vi "Execution Settings.vi"(8 "error in (no error)":errorcluster, 11 "Configuration in":refnum<class "Configuration.lvclass">) -> (0 "error out":errorcluster, 3 "Configuration out":refnum<class "Configuration.lvclass">)   [LabVIEW 2026, in "Measurement Actor.lvlib" / "Step Configuration.lvclass"]
uses:
  Step Configuration.lvclass
  Extensible-Config-Dialog/Configuration.lvclass
  C:/Users/E2013170/Documents/GitHub/Measurement-Utility-Reference/components/Extensible-Config-Dialog/Configuration.lvclass
  Step Configuration.lvclass/Step Configuration.ctl
panel:
  in  "Execution Settings":T1
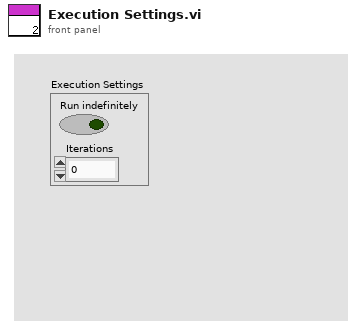
[diagram p1: front panel]
types:
  T1 = cluster{"Run indefinitely":bool, "Iterations":dbl}
  T2 = cluster{"Run indefinitely":bool, "Iterations":i32}
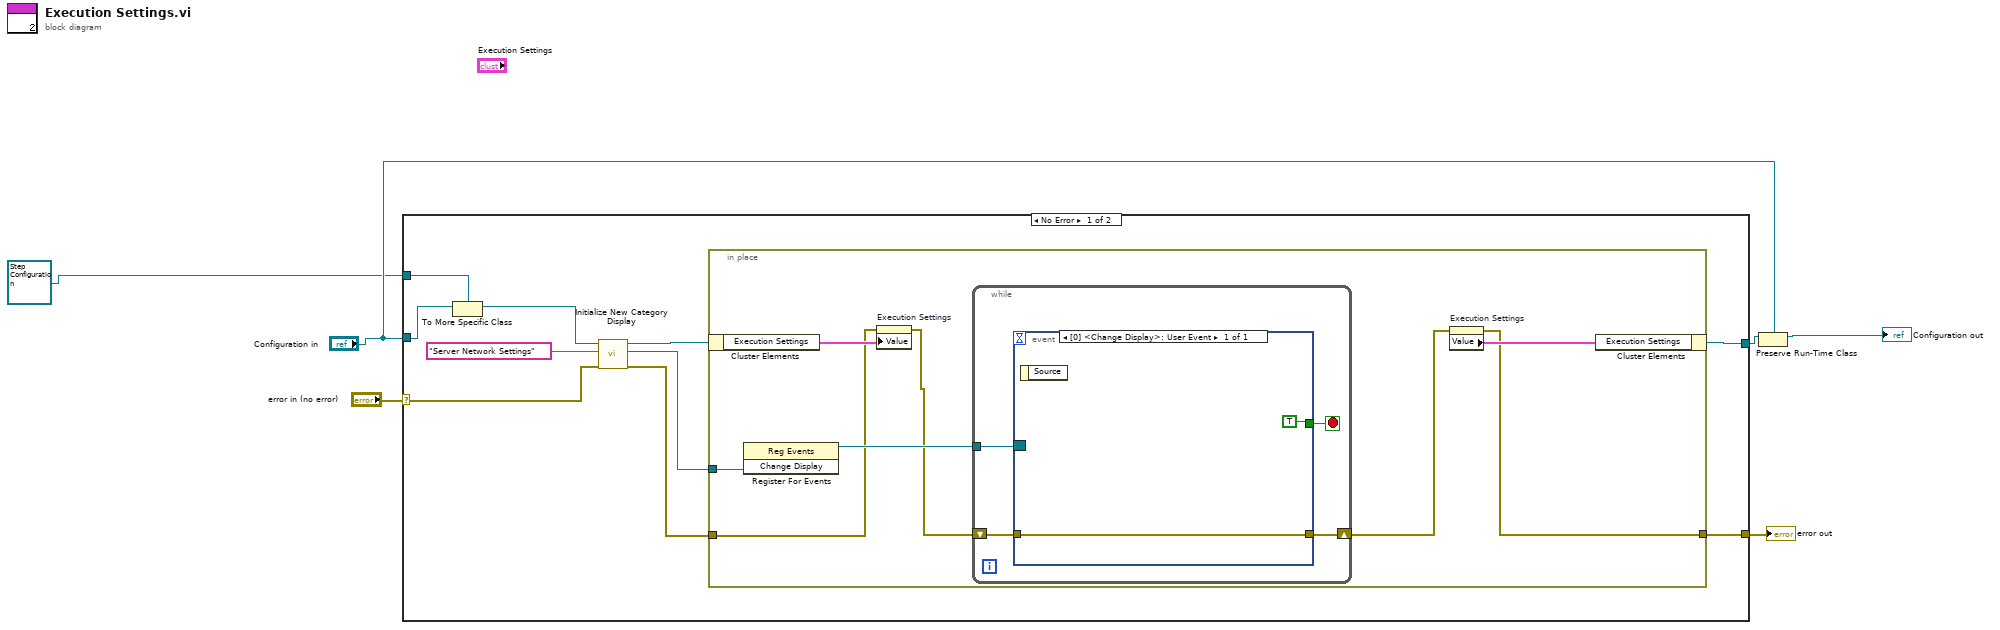
[diagram p0: block diagram]
diagram:
  n1 = case shown="No Error" "error in (no error)" {
    selector: "error in (no error)" -> [w13 w32]
    tunnel: [w12 w31] -> w3
    tunnel: [w7 w32] -> w6
    tunnel: "Configuration in" -> [w10 w31]
    tunnel: refnum<class "Step Configuration.lvclass"> refnum ("Measurement Actor.lvlib:Step Configuration.lvclass") -> [w8 _]
    frame No Error {
      n2 = To More Specific Class(target class=w8, reference=w10) -> (specific class reference=w9:refnum<class "Step Configuration.lvclass">)  [unwired: 1 in, 1 out]
      n3 = call "Initialize New Category Display.vi"("error in (no error)"=w13, "Name to Display"="Server Network Settings", "Configuration in"=w9) -> ("error out"=w15:errorcluster, "Change Display"=w16:refnum<user-event>, "Configuration Out"=w11:refnum<class "Step Configuration.lvclass">)  [unwired: 6 in]
      n4 = in-place {
        in-place-border: w16 -> [w24]
        in-place-border: w15 -> [w21]
        in-place-border: [w17] -> w7
        n5 = in-place-cluster #1(w11) -> ("Execution Settings"=w22:T2)
        n6 = register-events(w24) -> (reference out=w23:refnum<event-registration>)  [unwired: 2 in, 1 out]
        n7 = property on="Execution Settings" class="Clust (strict)"(error in=w21, "Value"=w22) -> (error out=w20:errorcluster)  [unwired: 1 in, 1 out]
        n8 = while {
          tunnel: w23 -> [w27]
          shift-right: [w26] -> w18
          shift-left: w20 -> [w25]
          stop <- w28 stop-if-true
          n9 = event shown="[0] <Change Display>: User Event" {
            selector: w27 -> [_]
            dyn-events: _ -> [_]
            timeout: _ -> [_]
            tunnel: [TRUE] -> w28
            tunnel: [w29] -> w26
            tunnel: w25 -> [w29]
            event User Event {
              n10 = event-data() -> ()  [unwired: 1 in, 1 out]
            }
          }
        }
        n11 = property on="Execution Settings" class="Clust (strict)"(error in=w18) -> (error out=w17:errorcluster, "Value"=w19:T1)  [unwired: 1 in, 1 out]
        n12 = in-place-cluster #1("Execution Settings"=w19) -> (w12:refnum<class "Step Configuration.lvclass">)
      }
    }
    frame Error {
    }
  }
  "error out" <- w6
  n13 = Preserve Run-Time Class(object in=w3, 2:"Configuration in") -> (object out=→"Configuration out":refnum<class "Configuration.lvclass">)  [unwired: 1 in, 1 out]
